vi "Run Offline Judge.vi"() -> ()   [LabVIEW 2014]
uses:
  Main Contest/Problem.ctl
panel:
  out "Status":string
  in  "TestCases Folder":path=path "C:/Users/Justin/Desktop/LabVIEW-Rank/Offline Judge/TestCases"
  in  "Problem":T1
  out "Accept?":bool
  # "You MUST have the path to the TestCases Folder entered before any tests can be run"
  # "Set this to the Correct Path"
  # "Open the Block Diagram and Place your VI in the box where it tells you to.\nUse the I/O terminals (found in the top-right) to create terminals for your VI.\nConnect these terminals tothe appropriate I/O of Offline Judge"
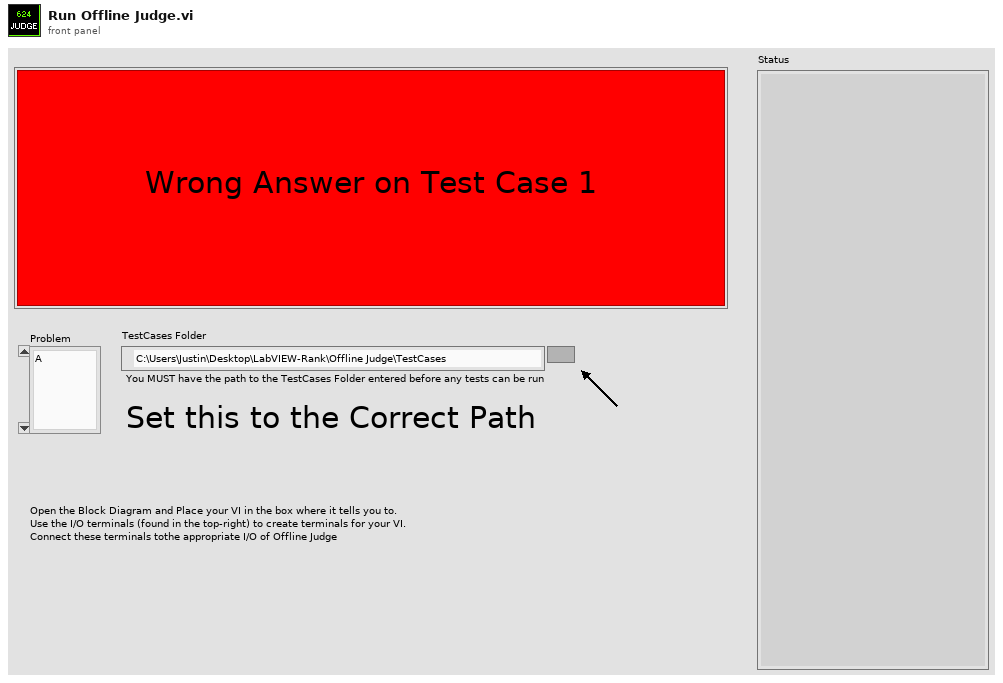
[diagram p1: front panel]
types:
  T1 = typedef "Problem.ctl" = enum16{"A", "B", "C", "D", "E"}
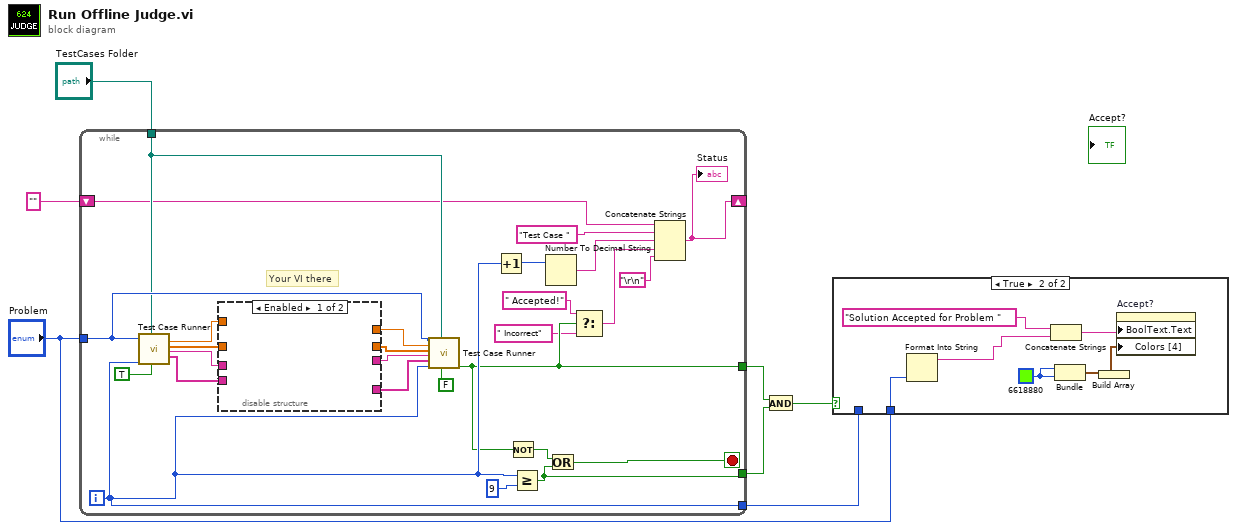
[diagram p0: block diagram]
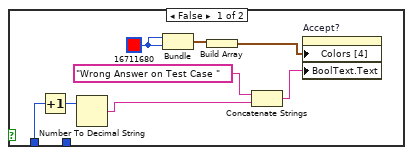
[diagram p2: hidden frame]
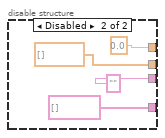
[diagram p3: hidden frame]
diagram:
  n1 = while {
    tunnel: "Problem" -> [w29]
    tunnel: [w31] -> w6
    tunnel: [w16] -> w5
    tunnel: [w12] -> w7
    tunnel: "TestCases Folder" -> [w19]
    shift-right: [w13] -> _
    shift-left: "" -> [w18]
    i -> [w16]
    stop <- w28 stop-if-true
    # "Your VI there"
    n2 = call "Test Case Runner.vi"("Problem"=w29, "Iterator"=w16, "TestCases Folder"=w19, "Send Input?"=TRUE ("Input")) -> ("Numeric"=w27:dbl, "Numeric Array"=w26:dbl[], "String"=w25:string, "String Array"=w24:string[])  [unwired: 11 in, 1 out]
    n3 = disable-structure shown="Enabled" {
      disable-tunnel: w27 -> [_ _]
      disable-tunnel: w26 -> [_ _]
      disable-tunnel: w25 -> [_ _]
      disable-tunnel: w24 -> [_ _]
      disable-tunnel: [_ 0.0 ("Numeric")] -> w23
      disable-tunnel: [_ dbl[] [] ("Numeric Array")] -> w22
      disable-tunnel: [_ "" ("String")] -> w21
      disable-tunnel: [_ string[] [] ("String Array")] -> w20
      frame Enabled {
      }
      frame Disabled {
      }
    }
    n4 = call "Test Case Runner.vi"("Problem"=w29, "Numeric 2"=w23, "Numeric Array 2"=w22, "String 2"=w21, "String Array 2"=w20, "Iterator"=w16, "TestCases Folder"=w19, "Send Input?"=FALSE) -> ("Accepted"=w12:bool)  [unwired: 7 in, 4 out]
    n5 = Increment(x=w16) -> (x+1=w15:i32)
    n6 = Not(x=w12) -> (.not. x?=w32:bool)
    n7 = Greater Or Equal?(x=w16, y=9) -> (x >= y?=w31:bool)
    n8 = Number To Decimal String(number=w15) -> (decimal integer string=w14:string)  [unwired: 1 in]
    n9 = Or(x=w32, y=w31) -> (x .or. y?=w28:bool)
    n10 = Select(t=" Accepted!", s=w12, f=" Incorrect") -> (s? t:f=w9:string)
    n11 = Concatenate Strings(w18, "Test Case ", w14, w9, "\r\n") -> (w13:string)
    "Status" <- w13
  }
  n12 = And(x=w7, y=w6) -> (x .and. y?=w4:bool)
  n13 = case shown="True" w4 {
    tunnel: w5 -> [w40 _]
    tunnel: "Problem" -> [_ w49]
    frame False {
      w45 = u32 16711680
      n14 = Increment(x=w40) -> (x+1=w39:i32)
      n15 = Number To Decimal String(number=w39) -> (decimal integer string=w41:string)  [unwired: 1 in]
      n16 = Bundle(w45, w45) -> (w46:cluster{u32, u32})  [unwired: 1 in]
      n17 = Build Array(w46) -> (w44:cluster{u32, u32}[])
      n18 = Concatenate Strings("Wrong Answer on Test Case " ("Boolean Text.Text"), w41) -> (w42:string)
      n19 = property on="Accept?" class="Bool (strict)"("Colors [4]"=w44, "BoolText.Text"=w42) -> ()  [unwired: 2 in, 2 out]
    }
    frame True {
      w53 = u32 6618880
      n20 = Format Into String(w49) -> (resulting string=w50:string)  [unwired: 3 in, 1 out]
      n21 = Concatenate Strings("Solution Accepted for Problem " ("Boolean Text.Text"), w50) -> (w47:string)
      n22 = Bundle(w53, w53) -> (w52:cluster{u32, u32})  [unwired: 1 in]
      n23 = Build Array(w52) -> (w51:cluster{u32, u32}[])
      n24 = property on="Accept?" class="Bool (strict)"("BoolText.Text"=w47, "Colors [4]"=w51) -> ()  [unwired: 2 in, 2 out]
    }
  }
